vi "custom.writer.vi"(5 "data":u8, 7 "data_valid":bool, 9 "end_of_frame":bool) -> (8 "niInstr Ethernet MAC Raw Stream v1.lvclass":refnum<class "niInstr Ethernet MAC Raw Stream v1.lvclass">)   [LabVIEW 2020]
uses:
  <instrlib>/_niInstr/Network/Ethernet/MAC/Raw Stream/v1/niInstr Ethernet MAC Raw Stream v1.lvclass
  <instrlib>/_niInstr/Network/Ethernet/Utility/v1/FPGA/Network Data Stream.ctl
  <instrlib>/_niInstr/Network/Ethernet/MAC/Raw Stream/v1/Write End of Good Frame.vi
  <instrlib>/_niInstr/Network/Ethernet/MAC/Raw Stream/v1/Write End of Bad Frame.vi
  <instrlib>/_niInstr/Network/Ethernet/MAC/Raw Stream/v1/Write Data Stream.vi
  <instrlib>/_niInstr/Network/Ethernet/Utility/v1/FPGA/niInstr Ethernet Utilities FPGA v1.lvlib
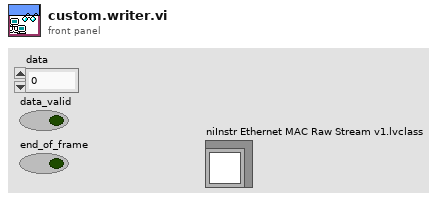
[diagram p1: front panel]
types:
  T1 = typedef "niInstr Ethernet Utilities FPGA v1.lvlib/Network Data Stream.ctl" = cluster{"data":u8[], "data valid":bool, "byte enables":bool[]}
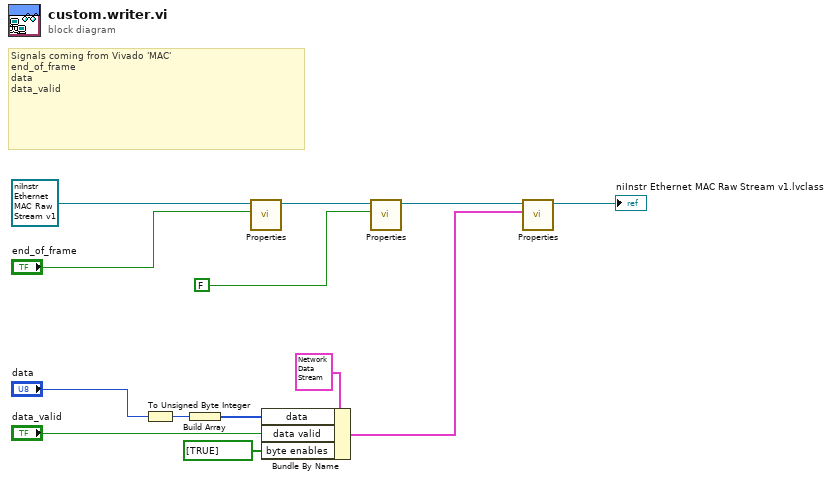
[diagram p0: block diagram]
diagram:
  # "Signals coming from Vivado 'MAC'\nend_of_frame\ndata\ndata_valid"
  n1 = To Unsigned Byte Integer(number="data") -> (unsigned 8bit integer=w10:u8)
  n2 = Build Array(w10) -> (w9:u8[])
  n3 = call-poly <instrlib>:"Properties.vi"("End of Good Frame"="end_of_frame", "niInstr Ethernet MAC Data Stream v1 in"=refnum<class "niInstr Ethernet MAC Raw Stream v1.lvclass"> refnum ("niInstr Ethernet MAC Metadata v1.lvclass")) -> ("niInstr Ethernet MAC Data Stream v1 out"=w13:refnum<class "niInstr Ethernet MAC Raw Stream v1.lvclass">)  [unwired: 9 in]
  n4 = Bundle By Name(cluster=T1 {"data"=[0, 0, 0, 0, 0, 0, 0, 0], "data valid"=FALSE, "byte enables"=[FALSE, FALSE, FALSE, FALSE, FALSE, FALSE, FALSE, FALSE]} ("Data Stream"), "data"=w9, "data valid"="data_valid", "byte enables"=bool[] [TRUE]) -> (w7:T1)
  n5 = call-poly <instrlib>:"Properties.vi"("End of Bad Frame"=FALSE, "niInstr Ethernet MAC Data Stream v1 in"=w13) -> ("niInstr Ethernet MAC Data Stream v1 out"=w12:refnum<class "niInstr Ethernet MAC Raw Stream v1.lvclass">)  [unwired: 9 in]
  n6 = call-poly <instrlib>:"Properties.vi"("Data Stream"=w7, "niInstr Ethernet MAC Data Stream v1 in"=w12) -> ("niInstr Ethernet MAC Data Stream v1 out"=→"niInstr Ethernet MAC Raw Stream v1.lvclass":refnum<class "niInstr Ethernet MAC Raw Stream v1.lvclass">)  [unwired: 9 in]
